vi "最大值判定.vi"(7 "Result":refnum<vi>, 10 "最大值判定":T1, 11 "XY曲线":cluster{"X":dbl[], "Y":dbl[]}[](array[cluster])) -> (2 "大小":i32, 3 "OK？":bool)   [LabVIEW 2020]
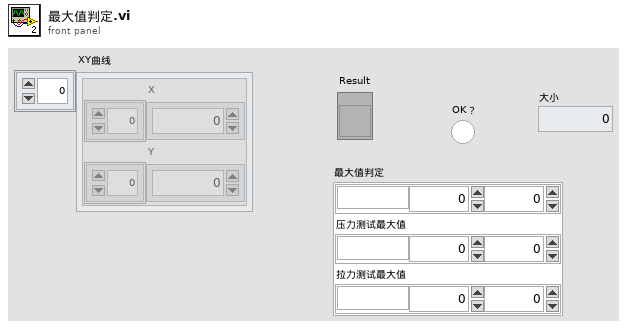
[diagram p1: front panel]
types:
  T1 = cluster{" 测试范围":cluster{"单位":string, "下限":dbl, "上限":dbl}, "压力测试最大值":cluster{"单位":string, "下限":dbl, "上限":dbl}, "拉力测试最大值":cluster{"单位":string, "下限":dbl, "上限":dbl}}
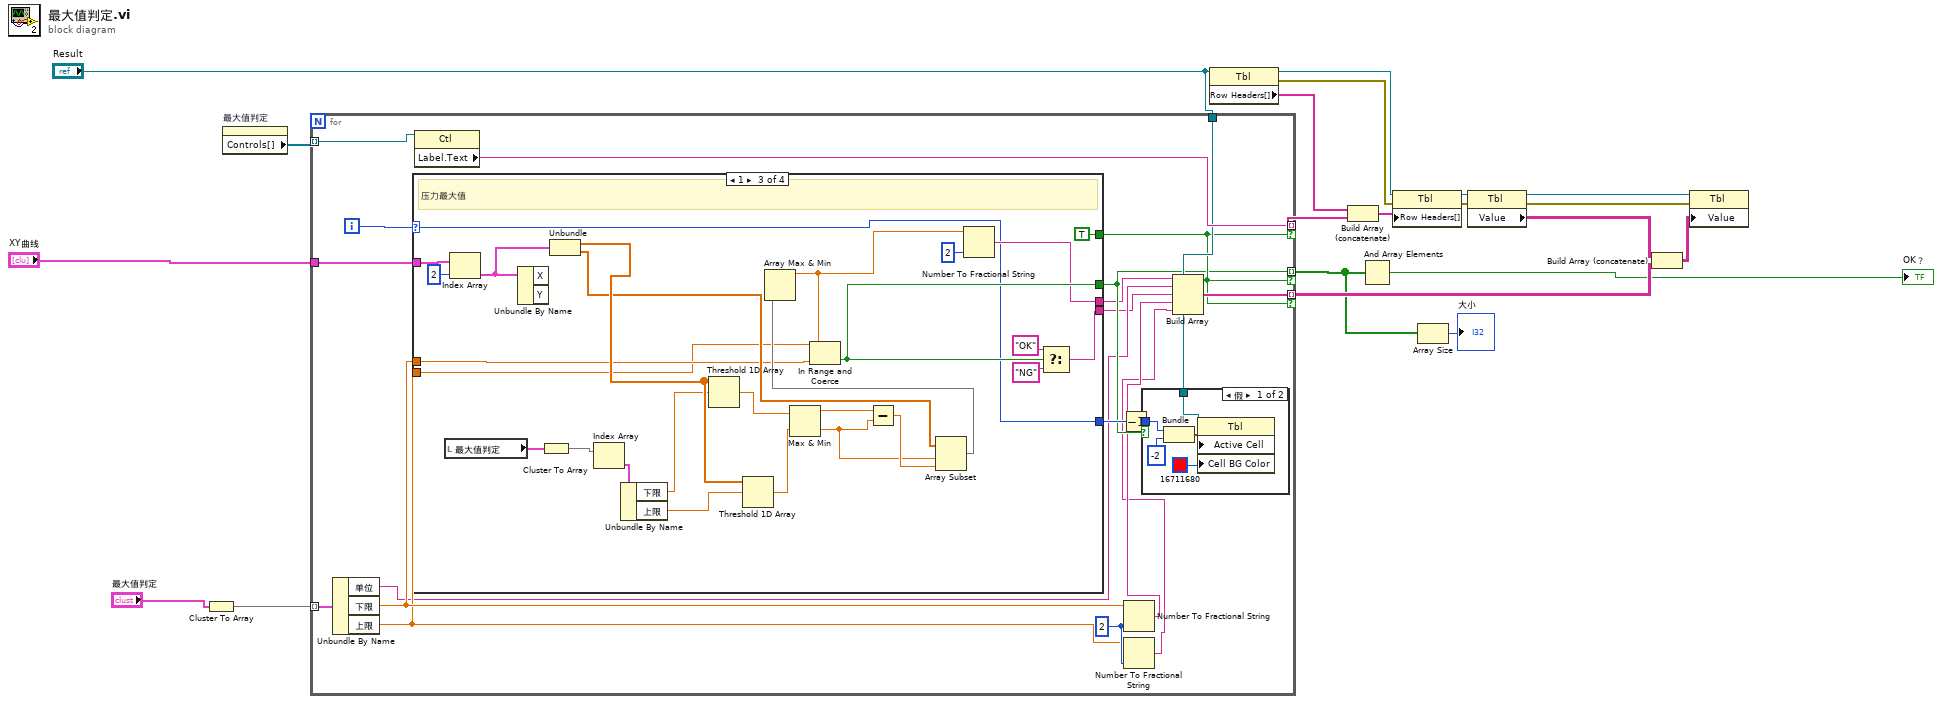
[diagram p0: block diagram]
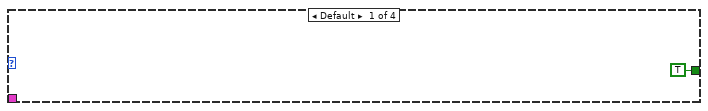
[diagram p3: hidden frame]
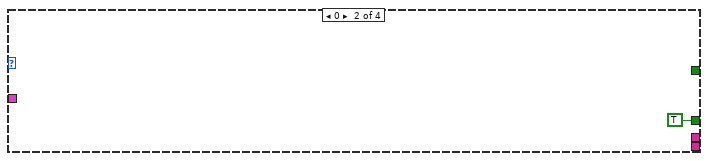
[diagram p4: hidden frame]
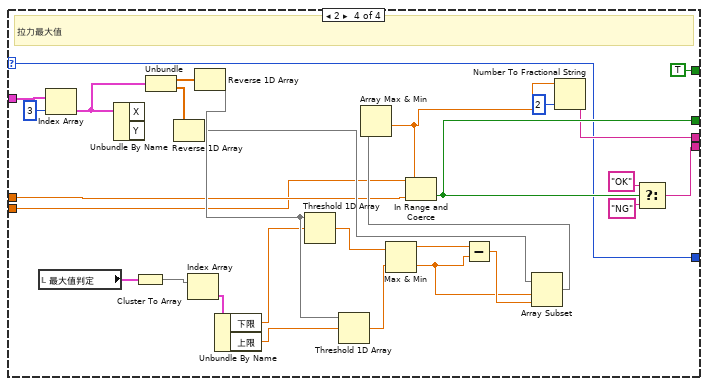
[diagram p5: hidden frame]
diagram:
  n1 = Cluster To Array(cluster="最大值判定") -> (array=w20:cluster{"单位":string, "下限":dbl, "上限":dbl}[])
  n2 = property on="最大值判定" class="Clust (严格)"() -> ("Controls[]"=w1:refnum<vi>[])  [unwired: 2 in, 2 out]
  n3 = for {
    tunnel: w20 -> [w39] mode=indexing
    tunnel: w1 -> [w37] mode=indexing
    tunnel: "XY曲线" -> [w36]
    tunnel: [w27] -> w3 mode=indexing if=w29
    tunnel: [w32] -> w7 mode=indexing if=w29
    tunnel: [w31] -> w9 mode=indexing if=w29
    tunnel: "Result" -> [w30]
    i -> [w38]
    w35 = i16 2 ("精度(6)")
    n4 = Unbundle By Name(w39) -> ("单位"=w25:string, "下限"=w34:dbl, "上限"=w33:dbl)
    n5 = case shown="1" w38 {
      selector: w38 -> [_ _ w54 w84]
      tunnel: w36 -> [_ _ w73 w102]
      tunnel: [_ _ w70 w99] -> w24
      tunnel: [_ TRUE w69 w98] -> w27
      tunnel: w34 -> [_ _ w53 w80]
      tunnel: w33 -> [_ _ w52 w79]
      tunnel: [TRUE _ TRUE TRUE] -> w29
      tunnel: [_ _ w55 w85] -> w26
      tunnel: [_ _ w54 w84] -> w28
      frame Default {
      }
      frame 0 {
      }
      frame 1 {
        # "压力最大值"
        n6 = local read "最大值判定"() -> (w51:T1)
        n7 = Index Array(array=w73, index=2 ("索引")) -> (element=w64:cluster{"X":dbl[], "Y":dbl[]})
        n8 = Unbundle By Name(w64) -> ()  [unwired: 2 out]
        n9 = Cluster To Array(cluster=w51) -> (array=w50:cluster{"单位":string, "下限":dbl, "上限":dbl}[])
        n10 = Unbundle(w64) -> ("X"=w63:dbl[], "Y"=w60:dbl[])
        n11 = Index Array(array=w50) -> (element=w49:cluster{"单位":string, "下限":dbl, "上限":dbl})  [unwired: 1 in]
        n12 = Unbundle By Name(w49) -> ("下限"=w48:dbl, "上限"=w47:dbl)
        n13 = Threshold 1D Array(2:w48, 3:w63) -> (0:w67:dbl)  [unwired: 1 in]
        n14 = Threshold 1D Array(2:w47, 3:w63) -> (0:w66:dbl)  [unwired: 1 in]
        n15 = Max & Min(x=w67, y=w66) -> (max(x,y)=w65:dbl, min(x,y)=w61:dbl)
        n16 = Subtract(x=w65, y=w61) -> (x-y=w62:dbl)
        n17 = Array Subset(array=w60, index=w61, length=w62) -> (w59:dbl[])
        n18 = Array Max & Min(array=w59) -> (max value=w56:dbl)  [unwired: 3 out]
        n19 = In Range and Coerce(upper limit=w52, x=w56, lower limit=w53) -> (In Range?=w69:bool)  [unwired: 1 out]
        n20 = Number To Fractional String(number=w56, precision (6)=i16 2 ("精度(6)")) -> (F-format string=w55:string)  [unwired: 2 in]
        n21 = Select(t="OK", s=w69, f="NG") -> (s? t:f=w70:string)
      }
      frame 2 {
        # "拉力最大值"
        n22 = local read "最大值判定"() -> (w78:T1)
        n23 = Index Array(array=w102, index=3 ("索引")) -> (element=w93:cluster{"X":dbl[], "Y":dbl[]})
        n24 = Unbundle By Name(w93) -> ()  [unwired: 2 out]
        n25 = Cluster To Array(cluster=w78) -> (array=w77:cluster{"单位":string, "下限":dbl, "上限":dbl}[])
        n26 = Unbundle(w93) -> ("X"=w92:dbl[], "Y"=w89:dbl[])
        n27 = Reverse 1D Array(array=w89) -> (reversed array=w82:dbl[])
        n28 = Index Array(array=w77) -> (element=w76:cluster{"单位":string, "下限":dbl, "上限":dbl})  [unwired: 1 in]
        n29 = Reverse 1D Array(array=w92) -> (reversed array=w83:dbl[])
        n30 = Unbundle By Name(w76) -> ("下限"=w75:dbl, "上限"=w74:dbl)
        n31 = Threshold 1D Array(2:w75, 3:w83) -> (0:w96:dbl)  [unwired: 1 in]
        n32 = Threshold 1D Array(2:w74, 3:w83) -> (0:w95:dbl)  [unwired: 1 in]
        n33 = Max & Min(x=w96, y=w95) -> (max(x,y)=w94:dbl, min(x,y)=w90:dbl)
        n34 = Subtract(x=w94, y=w90) -> (x-y=w91:dbl)
        n35 = Array Subset(array=w82, index=w90, length=w91) -> (w88:dbl[])
        n36 = Array Max & Min(array=w88) -> (min value=w87:dbl)  [unwired: 3 out]
        n37 = In Range and Coerce(upper limit=w79, x=w87, lower limit=w80) -> (In Range?=w98:bool)  [unwired: 1 out]
        n38 = Number To Fractional String(number=w87, precision (6)=i16 2 ("精度(6)")) -> (F-format string=w85:string)  [unwired: 2 in]
        n39 = Select(t="OK", s=w98, f="NG") -> (s? t:f=w99:string)
      }
    }
    n40 = property class="Ctl"(reference=w37) -> ("Label.Text"=w31:string)  [unwired: 1 in, 2 out]
    n41 = Decrement(x=w28) -> (x-1=w21:i32)
    n42 = Number To Fractional String(number=w34, precision (6)=w35) -> (F-format string=w23:string)  [unwired: 2 in]
    n43 = Number To Fractional String(number=w33, precision (6)=w35) -> (F-format string=w22:string)  [unwired: 2 in]
    n44 = case shown="假" w27 {
      tunnel: w30 -> [w44 _]
      tunnel: w21 -> [w40 _]
      frame False {
        n45 = Bundle(w40, -2) -> (w42:cluster{i32, i32})  [unwired: 1 in]
        n46 = property class="Tbl"(reference=w44, "Active Cell"=w42, "Cell BG Color"=u32 16711680 ("活动单元格:单元格背景色")) -> ()  [unwired: 1 in, 2 out]
      }
      frame True {
      }
    }
    n47 = Build Array(w26, w25, w24, w23, w22) -> (w32:string[])
  }
  n48 = property class="Tbl"(reference="Result") -> (reference out=w11:refnum<vi>, error out=w16:errorcluster, "Row Headers[]"=w8:string[])  [unwired: 1 in]
  n49 = Build Array (concatenate)(w8, w9) -> (w10:string[])
  n50 = And Array Elements(Boolean array=w3) -> (logical AND=→"OK？":bool)
  n51 = property class="Tbl"(reference=w11, error in=w16, "Row Headers[]"=w10) -> (reference out=w12:refnum<vi>, error out=w15:errorcluster)
  n52 = Array Size(array=w3) -> (size(s)=→"大小":i32)
  n53 = property class="Tbl"(reference=w12, error in=w15) -> (reference out=w13:refnum<vi>, error out=w14:errorcluster, "Value"=w17:string[][])
  n54 = Build Array (concatenate)(w17, w7) -> (w18:string[][])
  n55 = property class="Tbl"(reference=w13, error in=w14, "Value"=w18) -> ()  [unwired: 2 out]
